vi "Write Configuration.vi"(8 "error in (no error)":errorcluster, 10 "Switch Schedule":T1) -> (0 "error out":errorcluster)   [LabVIEW 2014]
uses:
  Controls/Switch Schedule.ctl
  Controls/Switch Program.ctl
  Controls/Action Enum.ctl
  Controls/Switch Day.ctl
  <vilib>/Utility/config.llb/Write Key (String).vi
  <vilib>/Utility/config.llb/NI_LVConfig.lvlib
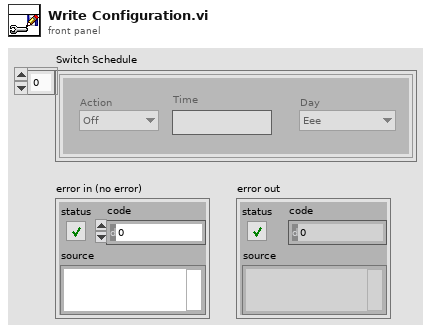
[diagram p1: front panel]
types:
  T1 = typedef "Switch Schedule.ctl" = T2[]
  T2 = typedef "Switch Program.ctl" = cluster{"Action":T3, "Time":string, "Day":T4}
  T3 = typedef "Action Enum.ctl" = enum16{"Off", "On"}
  T4 = typedef "Switch Day.ctl" = enum16{"Eee", "Sun", "Mon", "Tue", "Wed", "Thu", "Fri", "Sat"}
  T5 = typedef "NI_LVConfig.lvlib/Config Data RefNum.ctl" = refnum<k1>
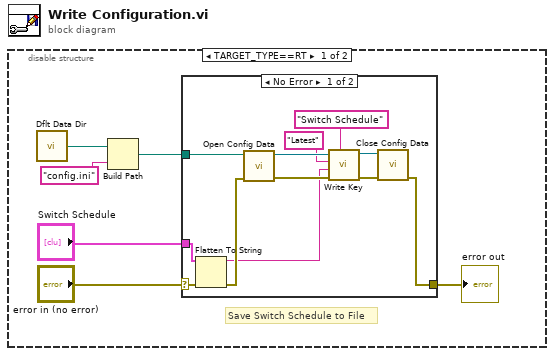
[diagram p0: block diagram]
diagram:
  n1 = disable-structure shown="TARGET_TYPE==RT" {
    frame condition #0 (active) {
      # "Save Switch Schedule to File"
      n2 = call <vilib>:"Dflt Data Dir.vi"() -> ("App:Default Data Directory"=w6:path)
      n3 = Build Path(base path=w6, name or relative path="config.ini") -> (appended path=w4:path)
      n4 = case shown="No Error" "error in (no error)" {
        selector: "error in (no error)" -> [w8 w19]
        tunnel: w4 -> [w18 _]
        tunnel: "Switch Schedule" -> [w17 _]
        tunnel: [w7 w19] -> w1
        frame No Error {
          n5 = Flatten To String(anything=w17, error in (no error)=w8) -> (data string=w11:string, error out=w16:errorcluster)  [unwired: 2 in, 1 out]
          n6 = call <vilib>:"Open Config Data.vi"("error in (no error)"=w16, "configuration file path"=w18) -> ("error out"=w14:errorcluster, "refnum"=w15:T5)  [unwired: 7 in, 1 out]
          n7 = call-poly <vilib>:"Write Key.vi"("section"="Switch Schedule", "error in (no error)"=w14, "value"=w11, "key"="Latest", "refnum"=w15) -> ("error out"=w10:errorcluster, "refnum out"=w9:T5)  [unwired: 4 in, 1 out]
          n8 = call <vilib>:"Close Config Data.vi"("error in (no error)"=w10, "refnum"=w9) -> ("error out"=w7:errorcluster)  [unwired: 8 in, 1 out]
        }
        frame Error {
        }
      }
      "error out" <- w1
    }
    frame condition #1 {
    }
  }
